vi "Do logging.vi"(0 "Critical Error":u8, 5 "Popup":string, 11 "error in (no error)":errorcluster) -> (4 "Numeric":u8, 15 "error out":errorcluster)   [LabVIEW 2020]
uses:
  Typedef's/Q_Operations.ctl
  Typedef's/Q_State.ctl
  <vilib>/SLL Toolkit/SLL String/_SubVIs/String to U8.vi
  <vilib>/SLL Toolkit/SLL String/SLL String.lvlib
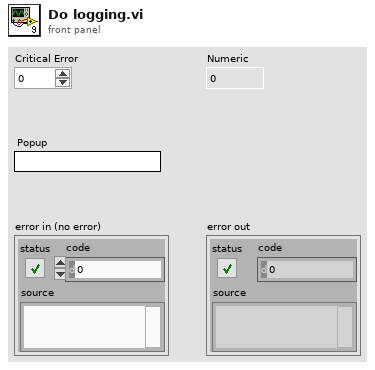
[diagram p1: front panel]
types:
  T1 = typedef "Q_State.ctl" = cluster{"State":string, "Data":variant}
  T2 = typedef "Q_Operations.ctl" = enum16{"Create Q", "Enqueue", "Dequeue", "Enqueue N ele", "Enstack N ele", "Flush Q", "Destroy Q"}
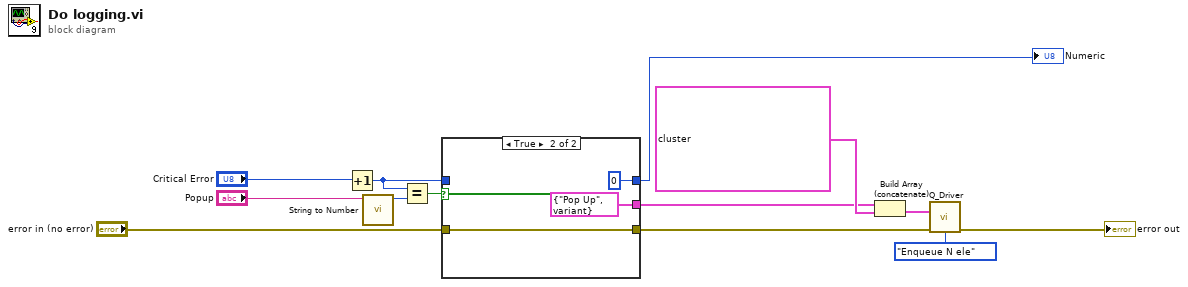
[diagram p0: block diagram]
diagram:
  n1 = Increment(x="Critical Error") -> (x+1=w7:u8)
  n2 = call-poly <vilib>:"String to Number.vi"("String"="Popup") -> ("Numeric"=w3:u8)  [unwired: 10 in]
  n3 = Equal?(x=w7, y=w3) -> (x = y?=w6:bool)
  n4 = case shown="True" w6 {
    tunnel: [w15 w18] -> w4
    tunnel: "error in (no error)" -> [w15 w18]
    tunnel: w7 -> [w14 _]
    tunnel: [w14 u8 0] -> w8
    tunnel: [_ T1 {"State"="Pop Up", "Data"=variant} ("State")] -> w9
    frame False {
    }
    frame True {
    }
  }
  "Numeric" <- w8
  n5 = Build Array (concatenate)(w9, T1[] [{"State"="Graph Updation", "Data"=variant}, {"State"="Description", "Data"=variant}, {"State"="Log Data Into Table", "Data"=variant}] ("appended array")) -> (w12:T1[])
  n6 = call "Q_Driver.vi"("States[]"=w12, "Error In"=w4, "Operations"=Q_Operations."Enqueue N ele") -> ("Error Out"=→"error out":errorcluster)  [unwired: 11 in, 1 out]
